vi "PCert-ConfigPageNF-Ask.vi"(6 "Timeout":i32=100 format="%dmsec", 8 "error in (no error)":errorcluster, 9 "Request Body":string, 10 "Request Header":string, 11 "ERP-ConfigPageNF in":refnum<class "PCert-ConfigPageNF.lvclass">) -> (0 "error out":errorcluster, 1 "Response Body":string, 2 "Response Header":string, 3 "ERP-ConfigPageNF out":refnum<class "PCert-ConfigPageNF.lvclass">)   [LabVIEW 2013, in "PCert-ConfigPageNF.lvclass"]
uses:
  PCert-ConfigPageNF.lvclass
  PCert-ConfigPageNF.lvclass/PCert-ConfigPageNF.ctl
  ftw-dataflow/Actor/src/Connector/FTW-ActorConnector.lvclass
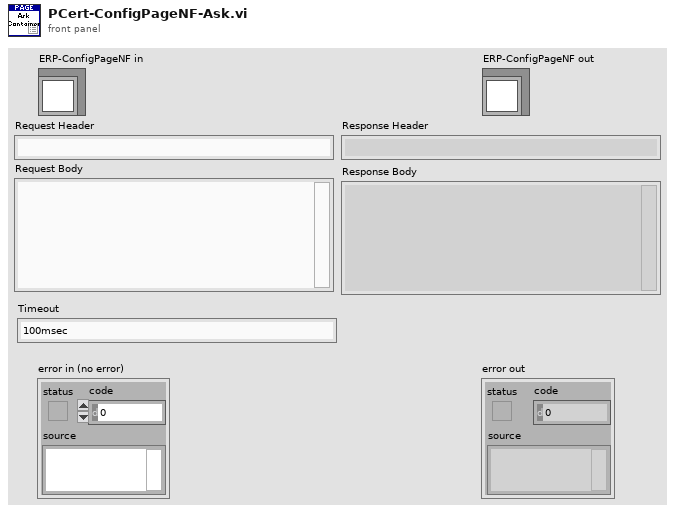
[diagram p1: front panel]
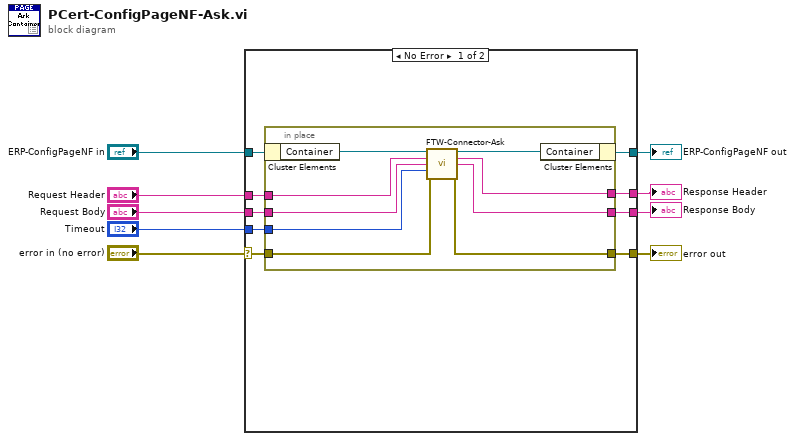
[diagram p0: block diagram]
diagram:
  n1 = case shown="No Error" "error in (no error)" {
    selector: "error in (no error)" -> [w17 w29]
    tunnel: [w16 w29] -> w8
    tunnel: [w12 w28] -> w6
    tunnel: "ERP-ConfigPageNF in" -> [w18 w28]
    tunnel: "Request Header" -> [w15 _]
    tunnel: "Request Body" -> [w14 _]
    tunnel: "Timeout" -> [w13 _]
    tunnel: [w11 _] -> w2
    tunnel: [w10 _] -> w1
    frame No Error {
      n2 = in-place {
        in-place-border: w17 -> [w25]
        in-place-border: [w24] -> w16
        in-place-border: w15 -> [w23]
        in-place-border: w14 -> [w22]
        in-place-border: w13 -> [w21]
        in-place-border: [w20] -> w11
        in-place-border: [w19] -> w10
        n3 = in-place-cluster #1(w18) -> ("Container"=w27:refnum<class "FTW-ActorConnector.lvclass">)
        n4 = call "FTW-Connector-Ask.vi"("FTW Actor Connector"=w27, "Request Header"=w23, "Request Body"=w22, "Timeout"=w21, "error in"=w25) -> ("FTW Actor Connector out"=w26:refnum<class "FTW-ActorConnector.lvclass">, "Response Header"=w20:string, "Response Body"=w19:string, "error out"=w24:errorcluster)  [unwired: 6 in, 1 out]
        n5 = in-place-cluster #1("Container"=w26) -> (w12:refnum<class "PCert-ConfigPageNF.lvclass">)
      }
    }
    frame Error {
    }
  }
  "error out" <- w8
  "ERP-ConfigPageNF out" <- w6
  "Response Header" <- w2
  "Response Body" <- w1
